vi "From Serial Form.vi"(8 "error in (no error)":errorcluster, 9 "Node":string, 10 "CI Deserializer in":refnum<class "CI Deserializer.lvclass">, 11 "Serializable Node in":refnum<class "Serializable Node.lvclass">) -> (0 "error out":errorcluster, 2 "CI Deserializer out":refnum<class "CI Deserializer.lvclass">, 3 "Serializable Node out":refnum<class "Serializable Node.lvclass">)   [LabVIEW 2014, in "Serializable Node.lvclass"]
uses:
  Serializable Node.lvclass
  CI Deserializer/CI Deserializer.lvclass
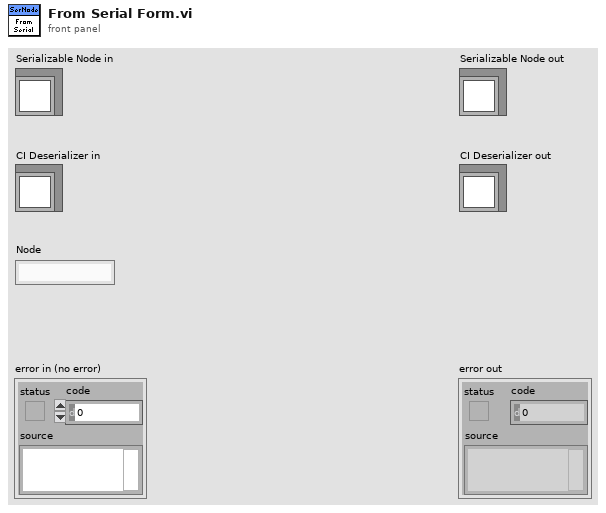
[diagram p1: front panel]
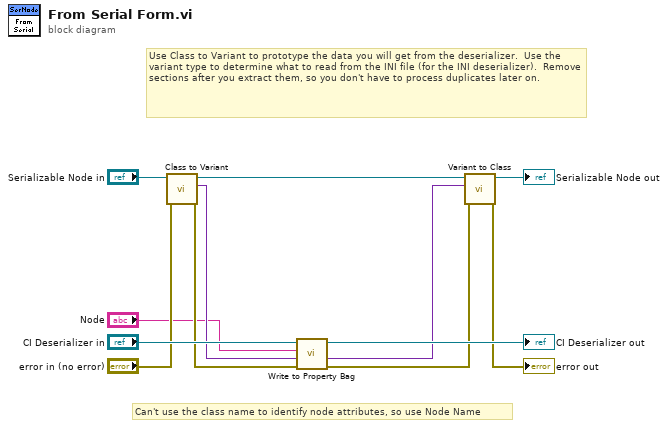
[diagram p0: block diagram]
diagram:
  # "Can't use the class name to identify node attributes, so use Node Name"
  # "Use Class to Variant to prototype the data you will get from the deserializer.  Use the variant type to determine what to read from the INI file (for the INI deserializer).  Remove sections after you extract them, so you don't have to process duplicates later on."
  n1 = call-dynamic "Class to Variant.vi"("error in (no error)"="error in (no error)", "Serializable Node in"="Serializable Node in") -> ("error out"=w2:errorcluster, "Data Out"=w3:variant, "Serializable Node out"=w10:refnum<class "Serializable Node.lvclass">)  [unwired: 6 in, 1 out]
  n2 = call-dynamic "Write to Property Bag.vi"("error in (no error)"=w2, "Prototype in"=w3, "Node"="Node", "CI Deserializer in"="CI Deserializer in") -> ("error out"=w6:errorcluster, "Data out"=w7:variant, "CI Deserializer out"=→"CI Deserializer out":refnum<class "CI Deserializer.lvclass">)  [unwired: 5 in]
  n3 = call-dynamic "Variant to Class.vi"("error in (no error)"=w6, "Data in"=w7, "Serializable Node in"=w10) -> ("error out"=→"error out":errorcluster, "Serializable Node out"=→"Serializable Node out":refnum<class "Serializable Node.lvclass">)  [unwired: 6 in, 1 out]
